vi "FPGA Sample Scanning V1.vi"() -> ()   [LabVIEW 2014]
uses:
  <vilib>/FPGAPlugInAG/PCIe-7852R/niLvFpga_Open_PCIe-7852R.vi
  <vilib>/FPGAPlugInAG/PCIe-7852R/niLvFpga_Reset_PCIe-7852R.vi
  <vilib>/Utility/error.llb/Error Cluster From Error Code.vi
  <vilib>/rvi/errors/niLvFpgaAdjustHostInterfaceError.vi
  <vilib>/FPGAPlugInAG/PCIe-7852R/niLvFpga_Run_PCIe-7852R.vi
  <vilib>/FPGAPlugInAG/PCIe-7852R/niLvFpga_Close_PCIe-7852R.vi
  <vilib>/rvi/interface/nirviOpenFPGA/nirviOpenFPGA.xnode
  FPGA Bitfiles/MainSTEDFPGAProj_FPGATarget2_StageScanningCam_oS-4DBWpl4s.lvbitx
  FPGA Target VIs/FPGA-7841R/Stage Scanning Cambridge V1.vi
  <vilib>/rvi/interface/nirviMethod/nirviMethod.xnode
  <vilib>/rvi/interface/nirviReadWriteControl/nirviReadWriteControl.xnode
  <vilib>/rvi/interface/nirviCloseFPGA/nirviCloseFPGA.xnode
  <vilib>/vision/NI_Vision_Development_Module.lvlib
  <vilib>/rvi/errors/niLvFpgaMergeErrorWithErrorCode.vi
  <vilib>/FPGAPlugInAG/PCIe-7852R/niLvFpga_ReadFifo_PCIe-7852R.vi
  NiFpgaLv.dll
  <vilib>/FPGAPlugInAG/PCIe-7852R/niLvFpga_StartFifo_PCIe-7852R.vi
panel:
  in  "Trigger Delay":u32=450000
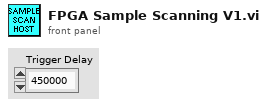
[diagram p1: front panel]
types:
  T1 = enum16{"big-endian, network order", "native, host order", "little-endian"}
  T2 = typedef "Scan Parameters.ctl" = cluster{"Fast_Ax_Amp_V":dbl, "Fast_Ax_Off_V":dbl, "Slow_Ax_Amp_V":dbl, "Slow_Ax_Off_V ":dbl, "Slow_Ax_Max_V_VperS":dbl, "Slow_Ax1_Del25ns":i32, "Slow_Ax2_Del25ns":i32, "Stage_X_Off_V":dbl, "Stage_Y_Off_V":dbl, "Stage_Z_Off_V":dbl, "Galvo1_Off_V":dbl, "Galvo2_Off_V":dbl, "Last_Scan_Mode":enum16{"XY", "XZ", "YZ", "XYZ"}, "Current_Scan_Mode":enum16{"XY", "XZ", "YZ", "XYZ"}, "Fly_Back_Lines":u16, "Linear_Ramp_End":u32, "Z_Step_I16":i16, "Z_Start_I16":i16, "Laser_States _U32":u32, "590_Voltage_I16":i16, "775_AOM_Volt_I16":i16, "Blanking OFF":bool, "Unused_Axis_I16":i16}
  T3 = typedef "Image Acquisition Parameters.ctl" = cluster{"Scan Type":enum16{"Sample Scanning", "Beam Scanning"}, "Scan Mode":enum16{"XY", "XZ", "YZ", "XYZ"}, "Fast Axis Frequency (Hz)":dbl, "Image Format":u16, "Line Accumulations":u16, "Frames Per Capture":u16, "Frames Accumulations":u16, "Image Dimension (um)":dbl[], "Number of Z Steps":u16, "Z Steps Size (um)":dbl, "Pixel Size (nm)":dbl[], "Customized Image Format":dbl[]}
  T4 = typedef "Detectors.ctl" = cluster{"PMT":bool, "Far Red (685/40 nm)":bool, "Orange (624/40 nm)":bool, "Green (525/50 nm)":bool, "Sum All":bool}
  T5 = typedef "IMAQ Image.ctl" = refnum<image>
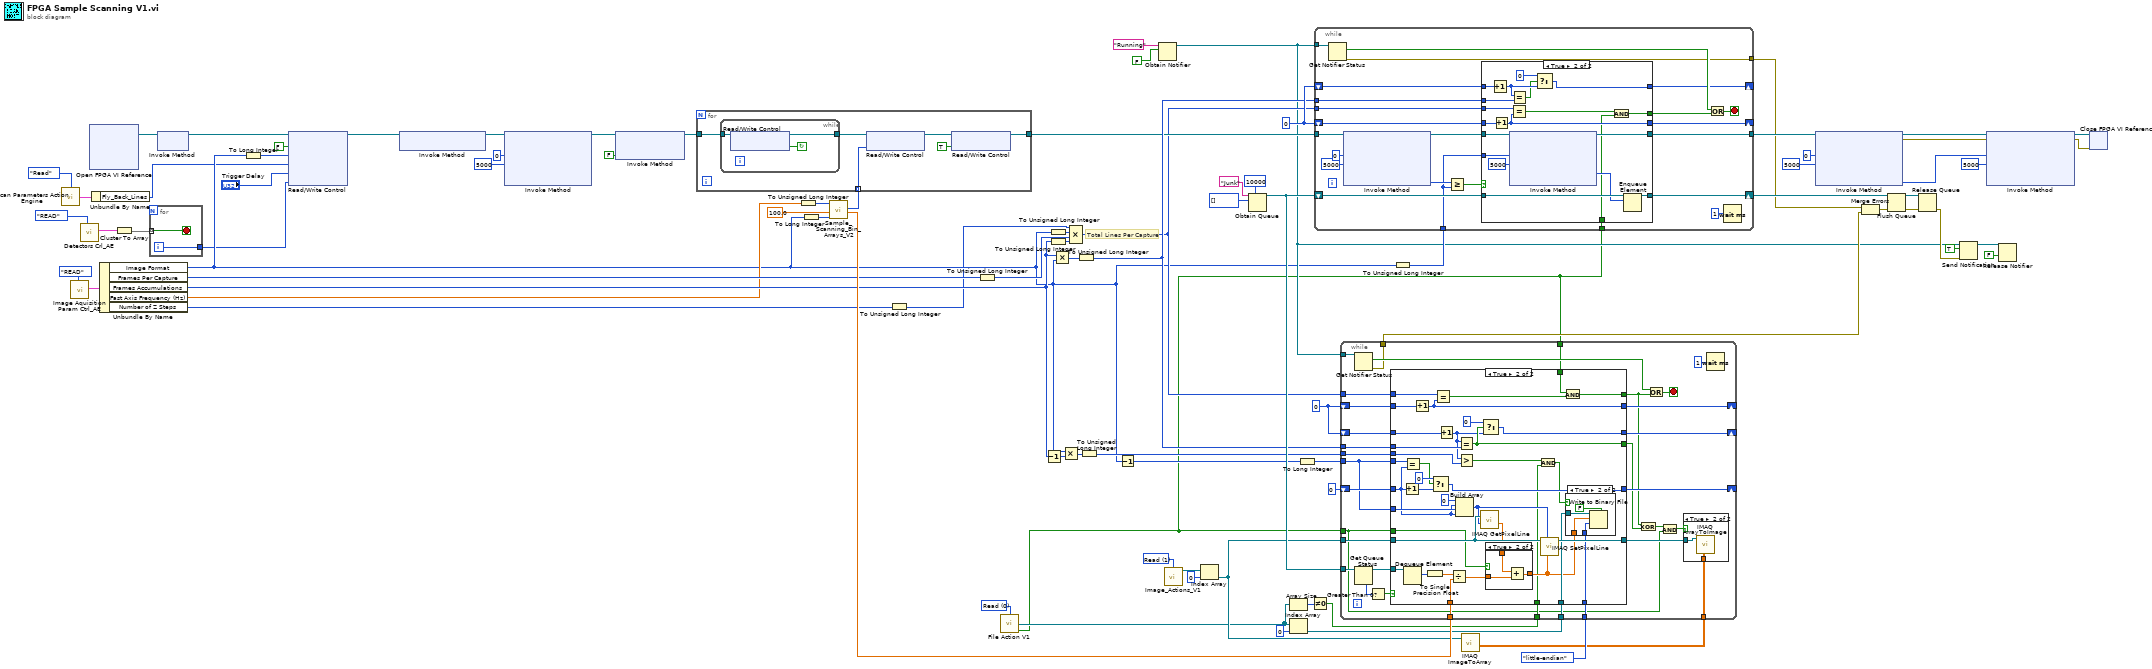
[diagram p0: block diagram]
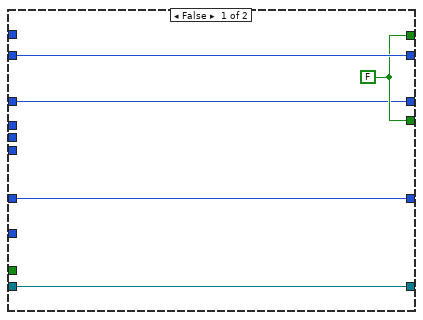
[diagram p3: hidden frame]
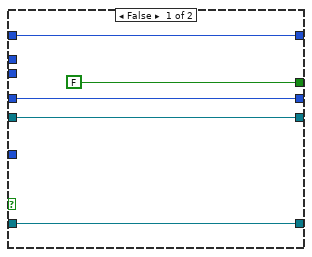
[diagram p6: hidden frame]
diagram:
  w24 = u16 0 items=["Read", "Write"] ("Mode")
  w27 = u32 0
  w32 = u16 1 items=["Write", "Read"] ("Mode")
  w63 = u32 0
  # "Total Lines Per Capture"
  n1 = call "Scan Parameters Action Engine.vi"("Action"=enum16{"Read", "Write"}."Read") -> ("Scan Parameters OUT"=w13:T2)  [unwired: 14 in]
  n2 = call "Image Aquisition Param Ctrl_AE.vi"("Action"=enum16{"READ", "WRITE"}."READ") -> ("Image Acquisition Parameters Out"=w5:T3)  [unwired: 10 in]
  n3 = call "Detectors Crl_AE.vi"("Action"=enum16{"READ", "WRITE"}."READ") -> ("Detectors Parameters Out"=w2:T4)  [unwired: 10 in]
  n4 = xnode "Open FPGA VI Reference"() -> ("FPGA VI Reference Out"=w38:refnum<k20>)  [unwired: 2 in, 1 out]
  n5 = Unbundle By Name(w13) -> ("Fly_Back_Lines"=w12:u16)
  n6 = Unbundle By Name(w5) -> ("Image Format"=w15:u16, "Frames Per Capture"=w48:u16, "Frames Accumulations"=w47:u16, "Fast Axis Frequency (Hz)"=w40:dbl, "Number of Z Steps"=w8:u16)
  n7 = Cluster To Array(cluster=w2) -> (array=w11:bool[])
  n8 = for {
    tunnel: w11 -> [w89] mode=indexing
    tunnel: [w88] -> w10
    i -> [w88]
    stop <- w89 stop-if-true
  }
  n9 = xnode "Invoke Method"("FPGA VI Reference In"=w38) -> ("FPGA VI Reference Out"=w37:refnum<k20>)  [unwired: 1 in, 1 out]
  n10 = To Long Integer(number=w15) -> (32bit integer=w42:i32)
  n11 = xnode "Read/Write Control"("FPGA VI Reference In"=w37, "Ready For Write"=FALSE, "Pixels Per Line"=w42, "Dead Lines"=w12, "Trigger Delay"="Trigger Delay", "APD Number"=w10) -> ("FPGA VI Reference Out"=w87:refnum<k20>)  [unwired: 1 in, 1 out]
  n12 = xnode "Invoke Method"("FPGA VI Reference In"=w87) -> ("FPGA VI Reference Out"=w86:refnum<k20>)  [unwired: 1 in, 1 out]
  n13 = xnode "Invoke Method"("FPGA VI Reference In"=w86, "Number of Elements"=u32 0, "Timeout (ms)"=5000) -> ("FPGA VI Reference Out"=w83:refnum<k20>)  [unwired: 1 in, 3 out]
  n14 = xnode "Invoke Method"("FPGA VI Reference In"=w83, "Wait Until Done (F)"=FALSE) -> ("FPGA VI Reference Out"=w60:refnum<k20>)  [unwired: 1 in, 1 out]
  n15 = To Unsigned Long Integer(number=w40) -> (unsigned 32bit integer=w17:u32)
  n16 = To Long Integer(number=w15) -> (32bit integer=w16:i32)
  n17 = call "Sample_Scanning_Bin_Arrays_V2.vi"("Pixels Per Line"=w16, "FPGA Acquisition Clock (MHz)"=100.0, "Scan Rate (Hz)"=w17) -> ("Normalization Array"=w54:sgl[], "Cycles Per Pixel"=w39:u32[])  [unwired: 3 in]
  n18 = for {
    tunnel: w60 -> [w95]
    tunnel: [w92] -> w57
    tunnel: w39 -> [w91] mode=indexing
    n19 = while {
      tunnel: w95 -> [w98]
      tunnel: [w96] -> w94
      stop <- w97 continue-if-true
      n20 = xnode "Read/Write Control"("FPGA VI Reference In"=w98) -> ("FPGA VI Reference Out"=w96:refnum<k20>, "Ready For Write"=w97:bool)  [unwired: 1 in, 1 out]
    }
    n21 = xnode "Read/Write Control"("FPGA VI Reference In"=w94, "Cycles Per Pixel"=w91) -> ("FPGA VI Reference Out"=w93:refnum<k20>)  [unwired: 1 in, 1 out]
    n22 = xnode "Read/Write Control"("FPGA VI Reference In"=w93, "Ready For Write"=TRUE ("Ready For Write (SLOW)")) -> ("FPGA VI Reference Out"=w92:refnum<k20>)  [unwired: 1 in, 1 out]
  }
  n23 = To Unsigned Long Integer(number=w8) -> (unsigned 32bit integer=w7:u32)
  n24 = To Unsigned Long Integer(number=w48) -> (unsigned 32bit integer=w46:u32)
  n25 = call "File Action V1.vi"("Mode"=w24) -> ("File REFs"=w22:refnum<file>[], "Files Open"=w9:bool)  [unwired: 12 in, 1 out]
  n26 = Decrement(x=w47) -> (x-1=w34:u16)
  n27 = To Unsigned Long Integer(number=w15) -> (unsigned 32bit integer=w68:u32)
  n28 = To Unsigned Long Integer(number=w47) -> (unsigned 32bit integer=w69:u32)
  n29 = Multiply(x=w47, y=w15) -> (x*y=w64:u16)
  n30 = Multiply(x=w15, y=w34) -> (x*y=w35:u16)
  n31 = Compound Arithmetic op=MULTIPLY(w7, w68, w46, w69) -> (w56:u32)
  n32 = To Unsigned Long Integer(number=w64) -> (unsigned 32bit integer=w62:u32)
  n33 = To Unsigned Long Integer(number=w35) -> (unsigned 32bit integer=w33:u32)
  n34 = Decrement(x=w15) -> (x-1=w36:u16)
  n35 = Obtain Notifier(name (unnamed)="Running", notification data type=FALSE) -> (notifier out=w43:refnum<notifier>)  [unwired: 2 in, 2 out]
  n36 = call "Image_Actions_V1.vi"("Mode"=w32) -> ("Image REFs OUT"=w30:T5[])  [unwired: 13 in, 1 out]
  n37 = Index Array(array=w30, index=0) -> (element=w29:T5)
  n38 = Obtain Queue(max queue size (-1, unlimited)=10000, name (unnamed)="Junk", element data type=u32[] []) -> (queue out=w70:refnum<queue>)  [unwired: 2 in, 2 out]
  n39 = Array Size(array=w22) -> (size(s)=w21:i32)
  n40 = Index Array(array=w22, index=0) -> (element=w20:refnum<file>)
  n41 = To Long Integer(number=w36) -> (32bit integer=w18:i32)
  n42 = Not Equal To 0?(x=w21) -> (x != 0?=w19:bool)
  n43 = To Unsigned Long Integer(number=w15) -> (unsigned 32bit integer=w67:u32)
  n44 = while {
    tunnel: w57 -> [w121]
    tunnel: [w117] -> w61
    tunnel: w67 -> [w109]
    tunnel: w43 -> [w113]
    shift-right: [w106] -> _
    shift-left: w63 -> [w108]
    tunnel: w56 -> [w107]
    shift-right: [w103] -> _
    shift-left: w63 -> [w104]
    tunnel: w62 -> [w102]
    tunnel: w9 -> [w101]
    tunnel: [w100] -> w50
    shift-right: [w115] -> w78
    shift-left: w70 -> [w116]
    stop <- w111 stop-if-true
    n45 = Get Notifier Status(notifier=w113) -> (current notification=w112:bool, error out=w100:errorcluster)  [unwired: 1 in, 3 out]
    n46 = xnode "Invoke Method"("FPGA VI Reference In"=w121, "Number of Elements"=u32 0, "Timeout (ms)"=5000) -> ("FPGA VI Reference Out"=w118:refnum<k20>, "Elements Remaining"=w114:u32)  [unwired: 1 in, 2 out]
    n47 = Greater Or Equal?(x=w114, y=w109) -> (x >= y?=w110:bool)
    n48 = case shown="True" w110 {
      tunnel: w118 -> [w126 w145]
      tunnel: w109 -> [_ w134]
      tunnel: [w126 w143] -> w117
      tunnel: w116 -> [w125 w142]
      tunnel: [w125 w141] -> w115
      tunnel: w108 -> [w124 w139]
      tunnel: w107 -> [_ w138]
      tunnel: [w124 w130] -> w106
      tunnel: [FALSE w128] -> w105
      tunnel: w104 -> [w123 w137]
      tunnel: [w123 w133] -> w103
      tunnel: w102 -> [_ w131]
      tunnel: w101 -> [_ w127]
      frame False {
      }
      frame True {
        n49 = Increment(x=w137) -> (x+1=w135:u32)
        n50 = Increment(x=w139) -> (x+1=w130:u32)
        n51 = xnode "Invoke Method"("FPGA VI Reference In"=w145, "Number of Elements"=w134, "Timeout (ms)"=5000) -> ("FPGA VI Reference Out"=w143:refnum<k20>, "Data"=w140:u64[])  [unwired: 1 in, 2 out]
        n52 = Equal?(x=w138, y=w130) -> (x = y?=w129:bool)
        n53 = Equal?(x=w135, y=w131) -> (x = y?=w132:bool)
        n54 = Select(t=u32 0, s=w132, f=w135) -> (s? t:f=w133:u32)
        n55 = And(x=w129, y=w127) -> (x .and. y?=w128:bool)
        n56 = Enqueue Element(queue=w142, element=w140) -> (queue out=w141:refnum<queue>)  [unwired: 2 in, 2 out]
      }
    }
    n57 = Or(x=w112, y=w105) -> (x .or. y?=w111:bool)
    n58 = Wait (ms)(milliseconds to wait=u32 1) -> ()  [unwired: 1 out]
  }
  n59 = call "IMAQ ImageToArray"("Image"=w29) -> ("Image Pixels (Float)"=w25:sgl[][])  [unwired: 3 in, 4 out]
  n60 = while {
    tunnel: w70 -> [w177]
    tunnel: w29 -> [w175]
    shift-right: [w173] -> _
    shift-left: 0 -> [w174]
    tunnel: w18 -> [w172]
    tunnel: w43 -> [w153]
    shift-right: [w167] -> _
    shift-left: w27 -> [w168]
    tunnel: w56 -> [w165]
    shift-right: [w161] -> _
    shift-left: w27 -> [w163]
    tunnel: w62 -> [w162]
    tunnel: w33 -> [w157]
    tunnel: T1."little-endian" ("byte order (0:big-endian, network order)") -> [w156]
    tunnel: w25 -> [w155]
    tunnel: w54 -> [w154]
    tunnel: w20 -> [w152]
    tunnel: w19 -> [w151]
    tunnel: [w150] -> w51
    tunnel: w9 -> [w149]
    tunnel: w9 -> [w146]
    stop <- w166 stop-if-true
    n61 = Get Notifier Status(notifier=w153) -> (current notification=w164:bool, error out=w150:errorcluster)  [unwired: 1 in, 3 out]
    n62 = Get Queue Status(queue=w177) -> (queue out=w176:refnum<queue>, # elements in queue=w171:i32)  [unwired: 2 in, 6 out]
    n63 = Greater Than 0?(x=w171) -> (x > 0?=w170:bool)
    n64 = case shown="True" w170 {
      tunnel: w176 -> [_ w221]
      tunnel: w175 -> [w183 w209]
      tunnel: w172 -> [_ w219]
      tunnel: w174 -> [w184 w214]
      tunnel: [w184 w215] -> w173
      tunnel: w172 -> [_ w216]
      tunnel: [w183 w213] -> w160
      tunnel: w168 -> [w182 w212]
      tunnel: [w182 w211] -> w167
      tunnel: [w181 w187] -> w158
      tunnel: w165 -> [_ w210]
      tunnel: [w181 w204] -> w159
      tunnel: w163 -> [w180 w202]
      tunnel: w162 -> [_ w205]
      tunnel: [w180 w203] -> w161
      tunnel: w157 -> [_ w200]
      tunnel: w156 -> [_ w199]
      tunnel: w152 -> [_ w198]
      tunnel: w154 -> [_ w194]
      tunnel: w151 -> [_ w189]
      tunnel: w149 -> [_ w186]
      tunnel: w146 -> [_ w185]
      frame False {
        w181 = FALSE
      }
      frame True {
        n65 = Increment(x=w214) -> (x+1=w217:i32)
        n66 = Dequeue Element(queue=w221) -> (element=w191:u32[])  [unwired: 2 in, 3 out]
        n67 = Equal?(x=w216, y=w214) -> (x = y?=w207:bool)
        n68 = Increment(x=w212) -> (x+1=w211:u32)
        n69 = To Single Precision Float(number=w191) -> (single precision float=w196:sgl[])
        n70 = Select(t=0, s=w207, f=w217) -> (s? t:f=w215:i32)
        n71 = Equal?(x=w210, y=w211) -> (x = y?=w188:bool)
        n72 = Increment(x=w202) -> (x+1=w201:u32)
        n73 = Divide(x=w196, y=w194) -> (x/y=w195:sgl[])
        n74 = Build Array(0, w214, w219, w214) -> (w208:i32[])
        n75 = Equal?(x=w201, y=w205) -> (x = y?=w204:bool)
        n76 = Greater?(x=w201, y=w200) -> (0:w190:bool)
        n77 = call "IMAQ GetPixelLine"("Line Coordinates"=w208, "Image"=w209) -> ("Pixels Line (Float)"=w197:sgl[])  [unwired: 2 in, 4 out]
        n78 = Select(t=u32 0, s=w204, f=w201) -> (s? t:f=w203:u32)
        n79 = case shown="True" w185 {
          tunnel: w197 -> [_ w225]
          tunnel: w195 -> [w222 w224]
          tunnel: [w222 w223] -> w193
          frame False {
          }
          frame True {
            n80 = Add(x=w225, y=w224) -> (x+y=w223:sgl[])
          }
        }
        n81 = And(x=w190, y=w189) -> (x .and. y?=w192:bool)
        n82 = call "IMAQ SetPixelLine"("Pixels Line (Float)"=w193, "Line Coordinates"=w208, "Image"=w209) -> ("Image Out"=w213:T5)  [unwired: 7 in, 1 out]
        n83 = And(x=w186, y=w188) -> (x .and. y?=w187:bool)
        n84 = case shown="True" w192 {
          tunnel: w193 -> [_ w226]
          tunnel: w199 -> [_ w228]
          tunnel: w198 -> [_ w227]
          frame False {
          }
          frame True {
            n85 = Write to Binary File(file (use dialog)=w227, data=w226, 5:FALSE ("prepend array or string size? (T)"), 9:w228) -> ()  [unwired: 2 in, 3 out]
          }
        }
      }
    }
    n86 = Exclusive Or(1:w159, 2:w158) -> (0:w148:bool)
    n87 = Or(x=w164, y=w158) -> (x .or. y?=w166:bool)
    n88 = And(x=w148, y=w146) -> (x .and. y?=w147:bool)
    n89 = case shown="True" w147 {
      tunnel: w160 -> [_ w179]
      tunnel: w155 -> [_ w178]
      frame False {
      }
      frame True {
        n90 = call "IMAQ ArrayToImage"("Image Pixels (Float)"=w178, "Image"=w179) -> ()  [unwired: 8 in, 2 out]
      }
    }
    n91 = Wait (ms)(milliseconds to wait=u32 1) -> ()  [unwired: 1 out]
  }
  n92 = xnode "Invoke Method"("FPGA VI Reference In"=w61, "Number of Elements"=u32 0, "Timeout (ms)"=5000) -> ("FPGA VI Reference Out"=w74:refnum<k20>, "error out"=w71:errorcluster, "Elements Remaining"=w73:u32)  [unwired: 1 in, 1 out]
  n93 = Merge Errors(w50, w51) -> (w66:errorcluster)
  n94 = Flush Queue(queue=w78, error in (no error)=w66) -> (queue out=w77:refnum<queue>, error out=w65:errorcluster)  [unwired: 1 out]
  n95 = Release Queue(queue=w77, error in (no error)=w65) -> (error out=w52:errorcluster)  [unwired: 1 in, 2 out]
  n96 = Send Notification(notification=TRUE, notifier=w43, error in (no error)=w52) -> (notifier out=w4:refnum<notifier>)  [unwired: 1 out]
  n97 = xnode "Invoke Method"("FPGA VI Reference In"=w74, "error in"=w71, "Number of Elements"=w73, "Timeout (ms)"=5000) -> ("FPGA VI Reference Out"=w59:refnum<k20>, "error out"=w58:errorcluster)  [unwired: 2 out]
  n98 = Release Notifier(notifier=w4, force destroy? (F)=FALSE) -> ()  [unwired: 1 in, 3 out]
  n99 = xnode "Close FPGA VI Reference"("FPGA VI Reference In"=w59, "error in"=w58) -> ()  [unwired: 1 out]
